vi "11-Alarm Management.vi"(8 "error in":errorcluster, 11 "ALID":u32) -> (0 "error out":errorcluster)   [LabVIEW 2020, in "SECS Scenarios.lvlib" / "Scenarios Class.lvclass"]
uses:
  Scenarios Class.lvclass
  11-Alarm Management.ctl
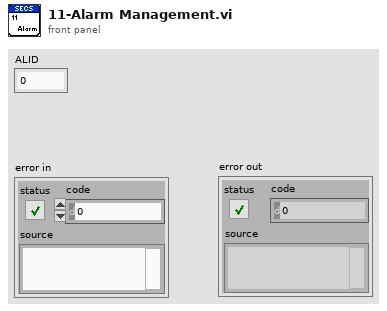
[diagram p1: front panel]
types:
  T1 = typedef "SECS Scenarios.lvlib/Scenarios Class.lvclass/11-Alarm Management.ctl" = cluster{"ALID":u32}
  T2 = typedef "SECS Scenarios.lvlib/Scenarios Class.lvclass/Request Refnum.ctl" = cluster{"11-Alarm Management":refnum<user-event>, "07-Event Report From Equipment":refnum<user-event>, "14-Process Program Creating Editing or Deleting":refnum<user-event>, "21-Material Movement":refnum<user-event>, "23-Equipment Sends Information to Host":refnum<user-event>, "24-Host Accepts On-Line Request from Equipment":refnum<user-event>, "25-Host Refuses On-Line Request":refnum<user-event>, "29-Equipment Requests Time Value from Host":refnum<user-event>, "33-Update Trace Data":refnum<user-event>}
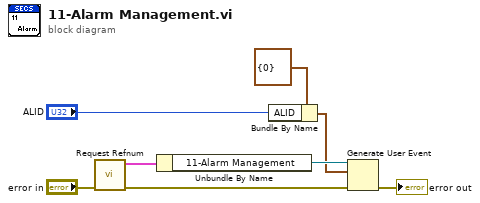
[diagram p0: block diagram]
diagram:
  n1 = call "Request Refnum.vi"("error in"="error in") -> ("error out"=w4:errorcluster, "Request Refnum"=w5:T2)  [unwired: 9 in]
  n2 = Unbundle By Name(w5) -> ("11-Alarm Management"=w3:refnum<user-event>)
  n3 = Bundle By Name(cluster=T1 {"ALID"=0} ("11-Alarm Management"), "ALID"="ALID") -> (w2:T1)
  n4 = Generate User Event(user event=w3, event data cluster=w2, error in=w4) -> (error out=→"error out":errorcluster)  [unwired: 1 in, 1 out]
